vi "Prepare_For_Consolidated_Save.vi"(7 "inside target file":bool, 8 "error in (no error)":errorcluster, 11 "AB_Source_VI in":refnum<class "AB_Source_VI.lvclass">) -> (0 "error out":errorcluster, 2 "item_Data":T1, 3 "AB_Source_VI out":refnum<class "AB_Source_VI.lvclass">)   [LabVIEW 2020, in "AB_Source_VI.lvclass"]
uses:
  <vilib>/AppBuilder/AB_Classes/Source/VI/AB_Source_VI.lvclass
  <vilib>/AppBuilder/Engine/AB_Engine_Consolidated_Save_Item_Info.ctl
  <vilib>/AppBuilder/AB_Classes/Source/VI/AB_Source_VI.lvclass/AB_Source_VI.ctl
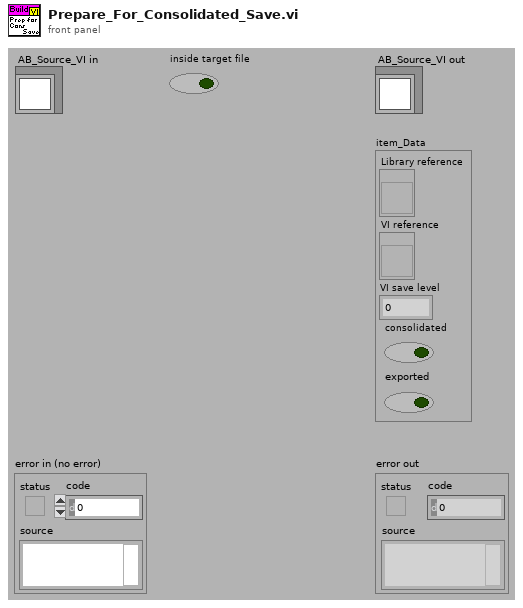
[diagram p1: front panel]
types:
  T1 = typedef "AB_Engine_Consolidated_Save_Item_Info.ctl" = cluster{"Library reference":refnum<vi>, "VI reference":refnum<vi>, "VI save level":i32, "consolidated":bool, "exported":bool}
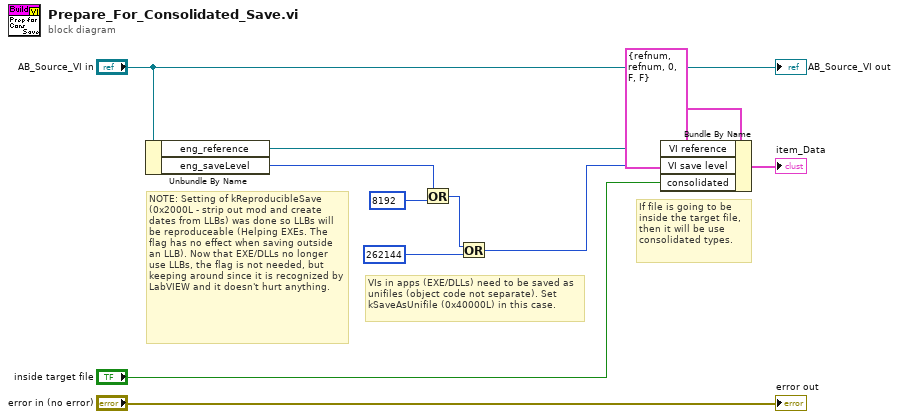
[diagram p0: block diagram]
diagram:
  # "If file is going to be inside the target file, then it will be use consolidated types."
  # "NOTE: Setting of kReproducibleSave (0x2000L - strip out mod and create dates from LLBs) was done so LLBs will be reproduceable (Helping EXEs. The flag has no effect when saving outside an LLB). Now that EXE/DLLs no longer use LLBs, the flag is not needed, but keeping around since it is recognized by LabVIEW and it doesn't hurt anything."
  # "VIs in apps (EXE/DLLs) need to be saved as unifiles (object code not separate). Set kSaveAsUnifile (0x40000L) in this case."
  n1 = Unbundle By Name("AB_Source_VI in") -> ("eng_reference"=w2:refnum<vi>, "eng_saveLevel"=w4:u32)
  n2 = Or(x=w4, y=u32 8192 ("data.eng_saveLevel")) -> (x .or. y?=w6:u32)
  n3 = Or(x=w6, y=u32 262144 ("data.eng_saveLevel")) -> (x .or. y?=w3:u32)
  n4 = Bundle By Name(cluster=T1 {"Library reference"=refnum, "VI reference"=refnum, "VI save level"=0, "consolidated"=FALSE, "exported"=FALSE} ("item_Data"), "VI reference"=w2, "VI save level"=w3, "consolidated"="inside target file") -> (→"item_Data":T1)
  "error out" <- "error in (no error)"
  "AB_Source_VI out" <- "AB_Source_VI in"
